vi "Przeładowanie mapy terenu.vi"(9 "Położenie startowe":cluster{"X [px]":i16, "Y [px]":i16}, 10 ">mapa z trasą robota>":picture, 11 "path to JPEG file":path) -> (0 "reload":bool, 1 "Nowe położenie  startowe [px]":cluster{"X [px]":i16, "Y [px]":i16}, 3 "Mapa terenu":picture)   [LabVIEW 2015, in "Biblioteka moduł map v3.lvlib" / "Obsługa grafiki mapy.lvlib"]
doc: "Modyfikacja pliku, który będzie nadpisywał wskazany plik jpg."
panel:
  out "Rectangle":T1
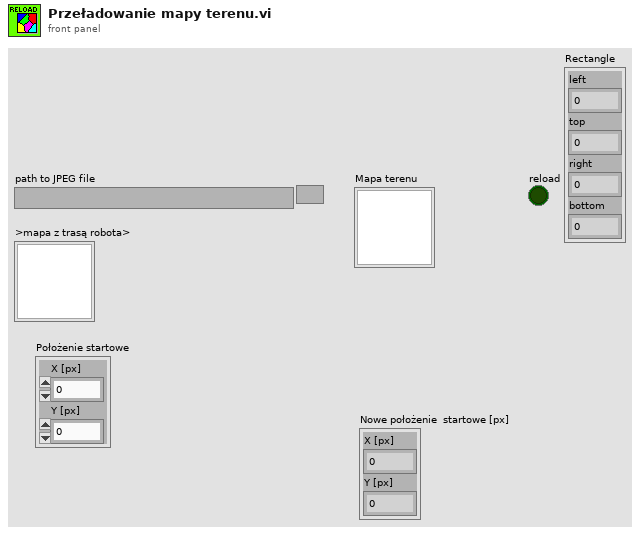
[diagram p1: front panel]
types:
  T1 = cluster{"left":i16, "top":i16, "right":i16, "bottom":i16}
  T2 = typedef "imagedata.ctl" = cluster{"image type":i32, "image depth":i32, "image":u8[], "mask":u8[], "colors":u32[], "Rectangle":cluster{"left":i16, "top":i16, "right":i16, "bottom":i16}}
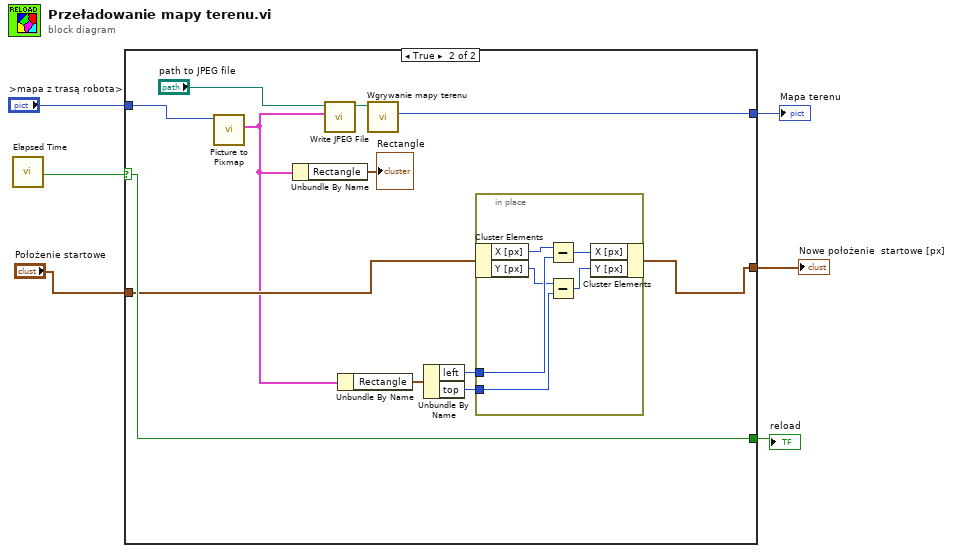
[diagram p0: block diagram]
diagram:
  n1 = call "Elapsed Time"() -> ("Time has Elapsed"=w1:bool)  [unwired: 12 in, 7 out]
  n2 = case shown="True" w1 {
    selector: w1 -> [w8 w18]
    tunnel: ">mapa z trasą robota>" -> [w9 w17]
    tunnel: [w9 w19] -> w6
    tunnel: [w8 w18] -> w4
    tunnel: "Położenie startowe" -> [w7 w12]
    tunnel: [w7 w10] -> w2
    frame False {
    }
    frame True {
      n3 = call <vilib>:"Picture to Pixmap.vi"("picture"=w17) -> ("image data"=w11:T2)  [unwired: 9 in, 1 out]
      n4 = Unbundle By Name(w11) -> ("Rectangle"=→"Rectangle":T1)
      n5 = call <vilib>:"Write JPEG File.vi"("image data"=w11, "path to JPEG file"="path to JPEG file") -> ("path"=w20:path)  [unwired: 8 in, 1 out]
      n6 = Unbundle By Name(w11) -> ("Rectangle"=w13:T1)
      n7 = call "Wgrywanie mapy terenu.vi"("Lokalizacja mapy terenu"=w20) -> ("Mapa terenu"=w19:picture)  [unwired: 9 in, 1 out]
      n8 = Unbundle By Name(w13) -> ("left"=w15:i16, "top"=w14:i16)
      n9 = in-place {
        in-place-border: w15 -> [w25]
        in-place-border: w14 -> [w24]
        n10 = in-place-cluster #1(w12) -> ("X [px]"=w27:i16, "Y [px]"=w23:i16)
        n11 = Subtract(x=w27, y=w25) -> (x-y=w26:i16)
        n12 = Subtract(x=w23, y=w24) -> (x-y=w22:i16)
        n13 = in-place-cluster #1("X [px]"=w26, "Y [px]"=w22) -> (w10:cluster{"X [px]":i16, "Y [px]":i16})
      }
    }
  }
  "Mapa terenu" <- w6
  "Nowe położenie  startowe [px]" <- w2
  "reload" <- w4
